vi "Using.vi"() -> ()   [LabVIEW 2010]
uses:
  St Using.ctl
panel:
  in  "Exit":bool
  in  "Stop":bool
  out "Slide":i32(slide) scale=0.0..2013.0
  out "Результат":i32
  in  "Діапазон":i32
  in  "Start":bool
  # "Випадкова генерація чисел"
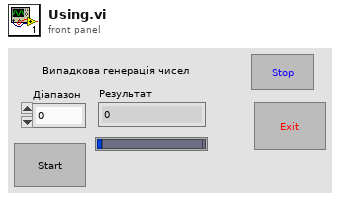
[diagram p1: front panel]
types:
  T1 = typedef "St Using.ctl" = enum16{"Start", "Stop", "Exit"}
  T2 = enum16{"Створ ч", "Зап на поч", "Зап на кін", "Зчит", "Очищ", "Видал"}
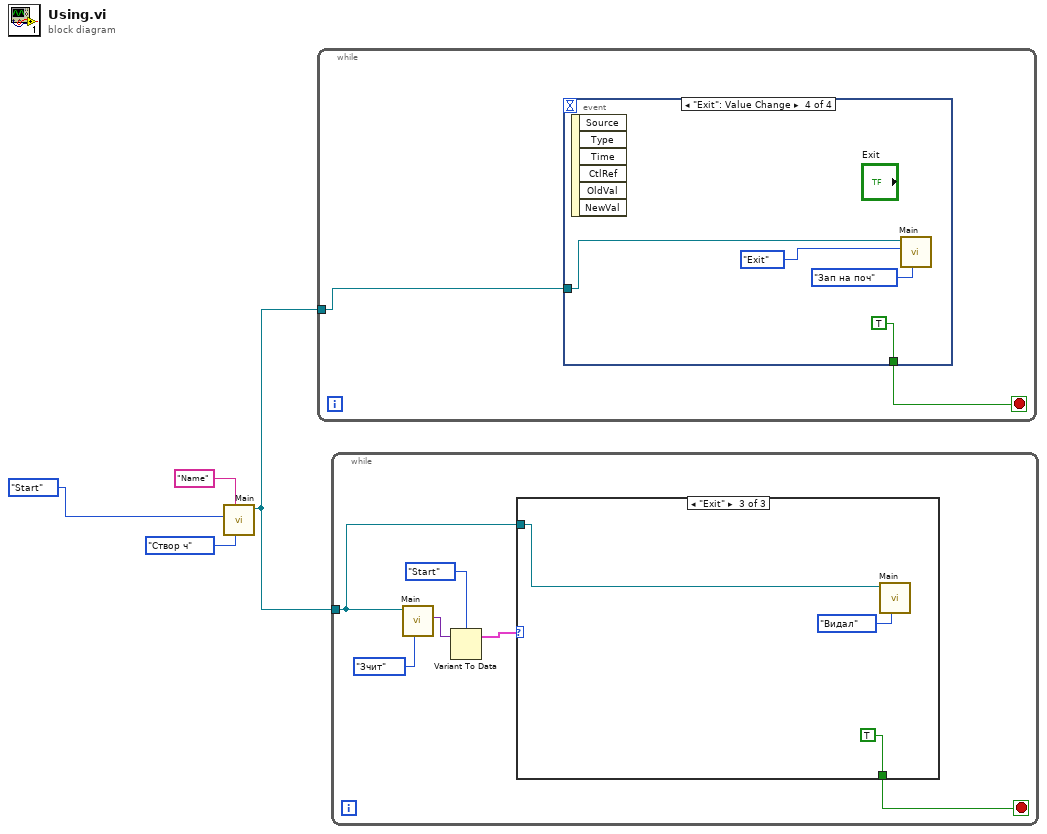
[diagram p0: block diagram]
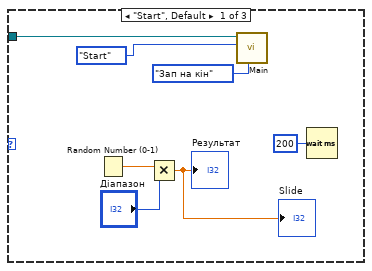
[diagram p2: hidden frame]
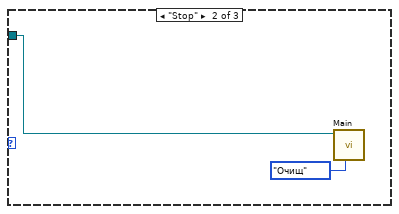
[diagram p3: hidden frame]
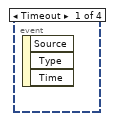
[diagram p4: hidden frame]
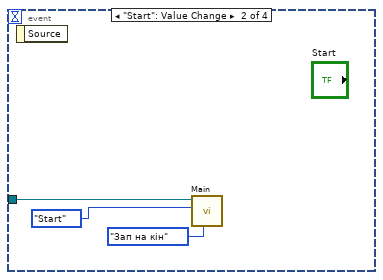
[diagram p5: hidden frame]
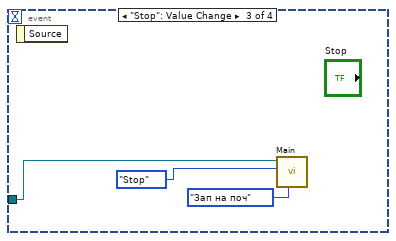
[diagram p6: hidden frame]
diagram:
  n1 = call "Main.vi"("States"=T2."Створ ч", "name"="Name", "elemint in"=St_Using."Start" ("Enum")) -> ("queue out"=w1:refnum<queue>)  [unwired: 4 in, 2 out]
  n2 = while {
    tunnel: w1 -> [w6]
    stop <- w5 stop-if-true
    n3 = event shown="[3] \"Exit\": Value Change" {
      selector: _ -> [_ _ _ _]
      dyn-events: _ -> [_ _ _ _]
      timeout: _ -> [_ _ _ _]
      tunnel: w6 -> [_ w8 w10 w13]
      tunnel: [_ _ _ TRUE] -> w5
      event Timeout {
        n4 = event-data() -> ()  [unwired: 1 in, 3 out]
      }
      event "Start": Value Change {
        n5 = event-data() -> ()  [unwired: 1 in, 1 out]
        n6 = call "Main.vi"("States"=T2."Зап на кін", "elemint in"=St_Using."Start" ("Enum"), "queue in"=w8) -> ()  [unwired: 4 in, 3 out]
      }
      event "Stop": Value Change {
        n7 = event-data() -> ()  [unwired: 1 in, 1 out]
        n8 = call "Main.vi"("States"=T2."Зап на поч", "elemint in"=St_Using."Stop" ("Enum"), "queue in"=w10) -> ()  [unwired: 4 in, 3 out]
      }
      event "Exit": Value Change {
        n9 = event-data() -> ()  [unwired: 1 in, 6 out]
        n10 = call "Main.vi"("States"=T2."Зап на поч", "elemint in"=St_Using."Exit" ("Enum"), "queue in"=w13) -> ()  [unwired: 4 in, 3 out]
      }
    }
  }
  n11 = while {
    tunnel: w1 -> [w18]
    stop <- w17 stop-if-true
    n12 = call "Main.vi"("States"=T2."Зчит", "queue in"=w18) -> ("element out"=w21:variant)  [unwired: 5 in, 2 out]
    n13 = Variant To Data(Variant=w21, type=St_Using."Start" ("Enum")) -> (data=w20:cluster{})  [unwired: 1 in, 1 out]
    n14 = case shown="\"Exit\"" w20 {
      tunnel: w18 -> [w25 w30 w33]
      tunnel: [_ _ TRUE] -> w17
      frame "Start", Default {
        n15 = Random Number (0-1)() -> (number: 0 to 1=w29:dbl)
        n16 = Multiply(x=w29, y="Діапазон") -> (x*y=→"Результат" →"Slide":dbl)
        n17 = call "Main.vi"("States"=T2."Зап на кін", "elemint in"=St_Using."Start" ("Enum"), "queue in"=w25) -> ()  [unwired: 4 in, 3 out]
        n18 = Wait (ms)(milliseconds to wait=u32 200) -> ()  [unwired: 1 out]
      }
      frame "Stop" {
        n19 = call "Main.vi"("States"=T2."Очищ", "queue in"=w30) -> ()  [unwired: 5 in, 3 out]
      }
      frame "Exit" {
        n20 = call "Main.vi"("States"=T2."Видал", "queue in"=w33) -> ()  [unwired: 5 in, 3 out]
      }
    }
  }
